vi "ClassExpansion.vi"(6 "ClassName Cache":refnum<data-value>, 8 "error in (no error)":errorcluster, 9 "expand objects on type conflict?":bool, 10 "To Object":refnum<class>, 11 "From Object":refnum<class>) -> (0 "error out":errorcluster, 2 "NumLevelsExpanded":u16, 3 "Target object":refnum<class>)   [LabVIEW 2020, in "BlueSerialization.lvlib" / "BlueSerializer.lvclass"]
uses:
  BlueSerializer.lvclass
  BlueSerializer.lvclass/BlueSerializer.ctl
  <vilib>/ErrorRing/Error Ring.xnode
  <vilib>/Utility/error.llb/Error Cluster From Error Code.vi
  ClassNameObj.ctl
  ClassNameCacheMap.ctl
  ClassNameCacheCluster.ctl
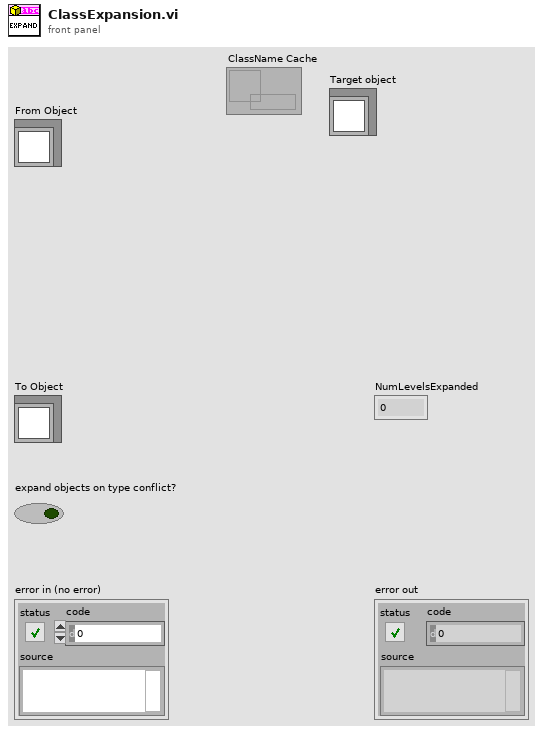
[diagram p1: front panel]
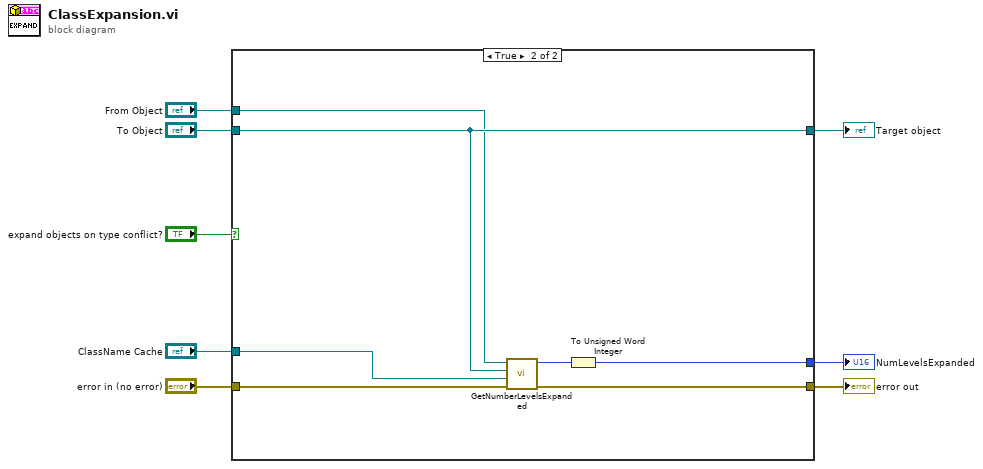
[diagram p0: block diagram]
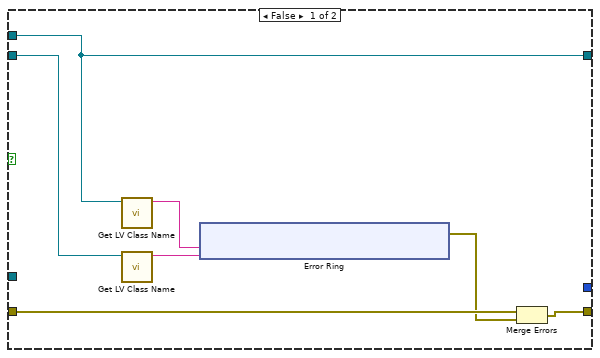
[diagram p2: hidden frame]
diagram:
  n1 = case shown="True" "expand objects on type conflict?" {
    tunnel: "To Object" -> [w13 w29]
    tunnel: [w15 w29] -> w1
    tunnel: "From Object" -> [w15 w28]
    tunnel: "error in (no error)" -> [w12 w25]
    tunnel: [w10 w24] -> w4
    tunnel: "ClassName Cache" -> [_ w26]
    tunnel: [_ w30] -> w2
    frame False {
      n2 = call <vilib>:"Get LV Class Name.vi"("object"=w15) -> ("class name"=w14:string)  [unwired: 9 in, 1 out]
      n3 = call <vilib>:"Get LV Class Name.vi"("object"=w13) -> ("class name"=w9:string)  [unwired: 9 in, 1 out]
      n4 = xnode "Error Ring"("parameter 0"=w14, "parameter 1"=w9) -> ("error out"=w11:errorcluster)
      n5 = Merge Errors(w12, w11) -> (w10:errorcluster)
    }
    frame True {
      n6 = call "GetNumberLevelsExpanded.vi"("error in (no error)"=w25, "ClassName Cache"=w26, "To object (more specific)"=w29, "From object (less specific)"=w28) -> ("error out"=w24:errorcluster, "NumLevelsExpanded"=w27:u32)  [unwired: 6 in]
      n7 = To Unsigned Word Integer(number=w27) -> (unsigned 16bit integer=w30:u16)
    }
  }
  "error out" <- w4
  "NumLevelsExpanded" <- w2
  "Target object" <- w1
